vi "PTScanner.form step list.vi"(2 "Sizes":i32[](array[numeric]), 3 "Object table":dbl[][](array[numeric])) -> (14 "Steps out":T2(array[cluster]))   [LabVIEW 2014, in "PTScanner.lvlib"]
uses:
  PTScanner.lvlib
  PTScanner.step obj parameters.ctl
panel:
  in  "Steps":T2(array[cluster])
  in  "Step":cluster{"Finished":bool, "object's setup":T1[]}
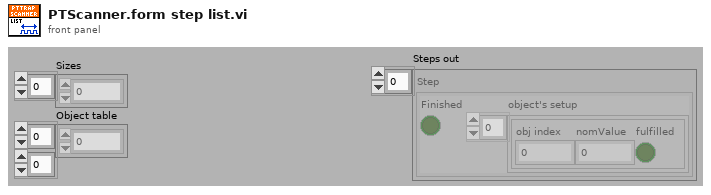
[diagram p1: front panel]
types:
  T1 = typedef "PTScanner.lvlib/PTScanner.step obj parameters.ctl" = cluster{"obj index":i32, "nomValue":dbl, "fulfilled":bool}
  T2 = cluster{"Finished":bool, "object's setup":T1[]}[]
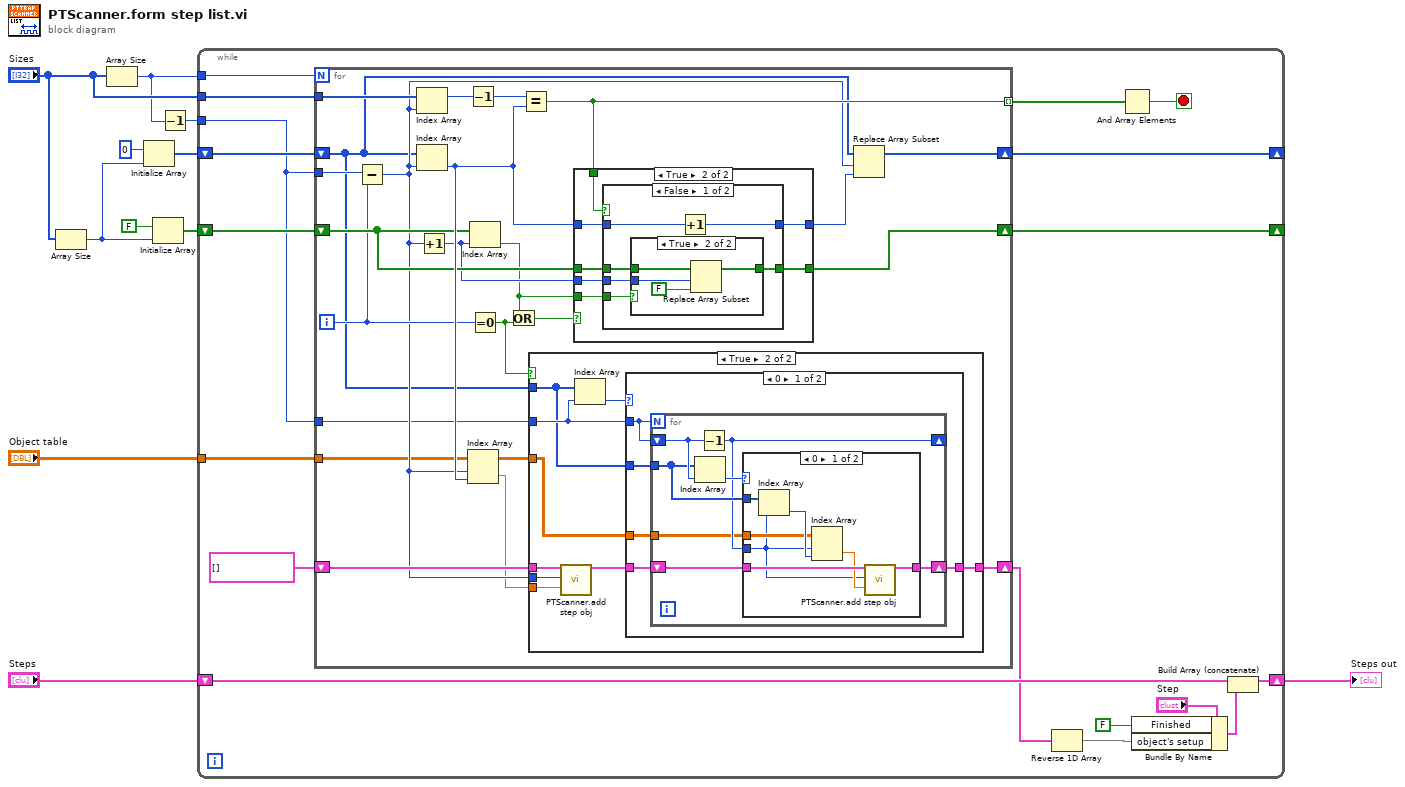
[diagram p0: block diagram]
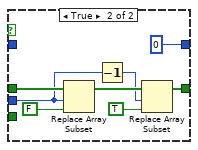
[diagram p7: hidden frame]
diagram:
  n1 = Array Size(array="Sizes") -> (size(s)=w3:i32)
  n2 = Array Size(array="Sizes") -> (size(s)=w2:i32)
  n3 = Initialize Array(0, w3) -> (w9:i32[])
  n4 = Initialize Array(FALSE, w3) -> (w8:bool[])
  n5 = Decrement(x=w2) -> (x-1=w1:i32)
  n6 = while {
    shift-right: [w23] -> _
    shift-left: w9 -> [w27]
    tunnel: "Object table" -> [w26]
    shift-right: [w17] -> w5
    shift-left: "Steps" -> [w25]
    shift-right: [w21] -> _
    shift-left: w8 -> [w22]
    tunnel: "Sizes" -> [w14]
    tunnel: w2 -> [w13]
    tunnel: w1 -> [w12]
    stop <- w28 stop-if-true
    n7 = for {
      N: w13 -> [_]
      tunnel: w14 -> [w50]
      tunnel: [w45] -> w29 mode=indexing
      tunnel: w26 -> [w31]
      tunnel: w12 -> [w49]
      shift-right: [w47] -> w23
      shift-left: w27 -> [w32]
      shift-right: [w40] -> w21
      shift-left: w22 -> [w42]
      shift-right: [w35] -> w15
      shift-left: T1[] [] ("Array") -> [w36]
      tunnel: w12 -> [w30]
      i -> [w38]
      n8 = Subtract(x=w49, y=w38) -> (x-y=w34:i32)
      n9 = Index Array(array=w50, index=w34) -> (element=w48:i32)
      n10 = Index Array(array=w32, index=w34) -> (element=w44:i32)
      n11 = Increment(x=w34) -> (x+1=w41:i32)
      n12 = Decrement(x=w48) -> (x-1=w51:i32)
      n13 = Index Array(array=w31, index (row)=w34, index (col)=w44) -> (element=w33:dbl)
      n14 = Index Array(array=w42, index=w41) -> (element=w39:bool)
      n15 = Equal To 0?(x=w38) -> (x = 0?=w37:bool)
      n16 = Or(x=w39, y=w37) -> (x .or. y?=w46:bool)
      n17 = Equal?(x=w51, y=w44) -> (x = y?=w45:bool)
      n18 = case shown="True" w37 {
        tunnel: w36 -> [w52 w61]
        tunnel: [w52 w56] -> w35
        tunnel: w34 -> [_ w60]
        tunnel: w33 -> [_ w59]
        tunnel: w32 -> [_ w54]
        tunnel: w31 -> [_ w53]
        tunnel: w30 -> [_ w55]
        frame False {
        }
        frame True {
          n19 = call "PTScanner.add step obj.vi"("array"=w61, "obj index"=w60, "nomValue"=w59) -> ("appended array"=w57:T1[])  [unwired: 16 in]
          n20 = Index Array(array=w54, index=w55) -> (element=w58:i32)
          n21 = case shown="0" w58 {
            tunnel: w57 -> [w64 w82]
            tunnel: [w63 w82] -> w56
            tunnel: w55 -> [w66 _]
            tunnel: w54 -> [w65 _]
            tunnel: w53 -> [w62 _]
            frame 0 {
              n22 = for {
                N: w66 -> [_]
                shift-right: [w68] -> _
                shift-left: w66 -> [w73]
                tunnel: w65 -> [w69]
                shift-right: [w70] -> w63
                shift-left: w64 -> [w71]
                tunnel: w62 -> [w67]
                n23 = Index Array(array=w69, index=w73) -> (element=w72:i32)
                n24 = Decrement(x=w73) -> (x-1=w68:i32)
                n25 = case shown="0" w72 {
                  tunnel: w71 -> [w77 w81]
                  tunnel: [w76 w81] -> w70
                  tunnel: w69 -> [w80 _]
                  tunnel: w68 -> [w74 _]
                  tunnel: w67 -> [w78 _]
                  frame 0 {
                    n26 = Index Array(array=w80, index=w74) -> (element=w79:i32)
                    n27 = Index Array(array=w78, index (row)=w74, index (col)=w79) -> (element=w75:dbl)
                    n28 = call "PTScanner.add step obj.vi"("array"=w77, "obj index"=w74, "nomValue"=w75) -> ("appended array"=w76:T1[])  [unwired: 16 in]
                  }
                  frame 1, Default {
                  }
                }
              }
            }
            frame 1, Default {
            }
          }
        }
      }
      n29 = case shown="True" w46 {
        tunnel: w45 -> [_ w91]
        tunnel: w44 -> [w84 w90]
        tunnel: [w84 w89] -> w43
        tunnel: w42 -> [w83 w88]
        tunnel: w41 -> [_ w87]
        tunnel: [w83 w86] -> w40
        tunnel: w39 -> [_ w85]
        frame False {
        }
        frame True {
          n30 = case shown="False" w91 {
            tunnel: w90 -> [w97 _]
            tunnel: [w96 0] -> w89
            tunnel: w88 -> [w95 w108]
            tunnel: w87 -> [w93 w105]
            tunnel: [w94 w103] -> w86
            tunnel: w85 -> [w92 _]
            frame False {
              n31 = case shown="True" w92 {
                tunnel: w95 -> [w98 w102]
                tunnel: w93 -> [_ w99]
                tunnel: [w98 w101] -> w94
                frame False {
                }
                frame True {
                  n32 = Replace Array Subset(array=w102, new element=FALSE, index=w99) -> (w101:bool[])
                }
              }
              n33 = Increment(x=w97) -> (x+1=w96:i32)
            }
            frame True {
              n34 = Replace Array Subset(array=w108, new element=FALSE, index=w105) -> (w109:bool[])
              n35 = Decrement(x=w105) -> (x-1=w104:i32)
              n36 = Replace Array Subset(array=w109, new element=TRUE, index=w104) -> (w103:bool[])
            }
          }
        }
      }
      n37 = Replace Array Subset(array=w32, new element=w43, index=w34) -> (w47:i32[])
    }
    n38 = Reverse 1D Array(array=w15) -> (reversed array=w18:T1[])
    n39 = And Array Elements(Boolean array=w29) -> (logical AND=w28:bool)
    n40 = Bundle By Name(cluster="Step", "Finished"=FALSE, "object's setup"=w18) -> (w19:cluster{"Finished":bool, "object's setup":T1[]})
    n41 = Build Array (concatenate)(w25, w19) -> (w17:T2)
  }
  "Steps out" <- w5
